vi "Init.vi"(8 "error in":errorcluster, 11 "IMAQdx Base Configure Strategy in":refnum<class "IMAQdx Base Configure Strategy.lvclass">) -> (0 "error out":errorcluster, 3 "IMAQdx Base Configure Strategy out":refnum<class "IMAQdx Base Configure Strategy.lvclass">)   [LabVIEW 2024, in "IMAQdx Base Configure Strategy.lvclass"]
uses:
  IMAQdx Base Configure Strategy.lvclass
  IMAQdx Base Configure Strategy.lvclass/IMAQdx Base Configure Strategy.ctl
  Source/Interfaces/IConfiguration/IConfiguration.lvclass
  <vilib>/vision/driver/NI_Vision_Acquisition_Software.lvlib
  <vilib>/vision/driver/IMAQdx.llb/IMAQdx Camera Control Mode.ctl
  <vilib>/userDefined/High Color/IMAQdx.ctl
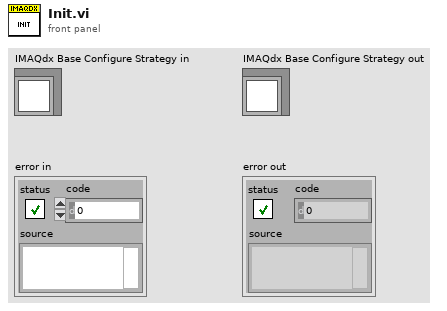
[diagram p1: front panel]
types:
  T1 = typedef "NI_Vision_Acquisition_Software.lvlib/IMAQdx Camera Control Mode.ctl" = enum32{"Controller", "Listener"}
  T2 = typedef "IMAQdx.ctl" = refnum<k21>
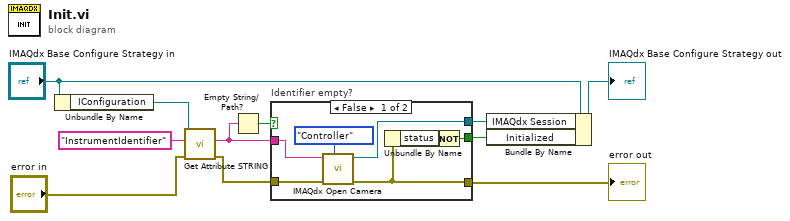
[diagram p0: block diagram]
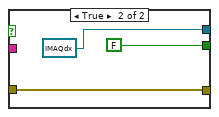
[diagram p2: hidden frame]
diagram:
  n1 = Unbundle By Name("IMAQdx Base Configure Strategy in") -> ("IConfiguration"=w10:refnum<class "IConfiguration.lvclass">)
  n2 = call-dynamic "Get Attribute STRING.vi"("error in"="error in", "Attribute"="InstrumentIdentifier", "IConfiguration in"=w10) -> ("error out"=w4:errorcluster, "Value"=w7:string)  [unwired: 6 in, 1 out]
  n3 = Empty String/Path?(string/path=w7) -> (empty?=w8:bool)
  n4 = case "Identifier empty?" shown="False" w8 {
    tunnel: [w14 w21] -> w5
    tunnel: [w16 T2 refnum ("Session Out")] -> w2
    tunnel: w7 -> [w15 _]
    tunnel: w4 -> [w18 w21]
    tunnel: [w12 FALSE] -> w1
    frame False {
      n5 = call <vilib>:"IMAQdx Open Camera.vi"("Camera Control Mode"=IMAQdx_Camera_Control_Mode."Controller", "error in"=w18, "Session In"=w15) -> ("error out"=w14:errorcluster, "Session Out"=w16:T2)  [unwired: 7 in]
      n6 = Unbundle By Name(w14) -> ("status"=w13:bool)
      n7 = Not(x=w13) -> (.not. x?=w12:bool)
    }
    frame True {
    }
  }
  "error out" <- w5
  n8 = Bundle By Name(cluster="IMAQdx Base Configure Strategy in", "IMAQdx Session"=w2, "Initialized"=w1) -> (→"IMAQdx Base Configure Strategy out":refnum<class "IMAQdx Base Configure Strategy.lvclass">)
